vi "div3sum-tsk3.vi"() -> ()   [LabVIEW 2020]
panel:
  out "Numeric":dbl
  out "quotient":dbl
  out "remainder":dbl
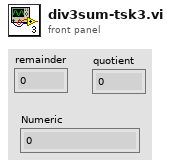
[diagram p1: front panel]
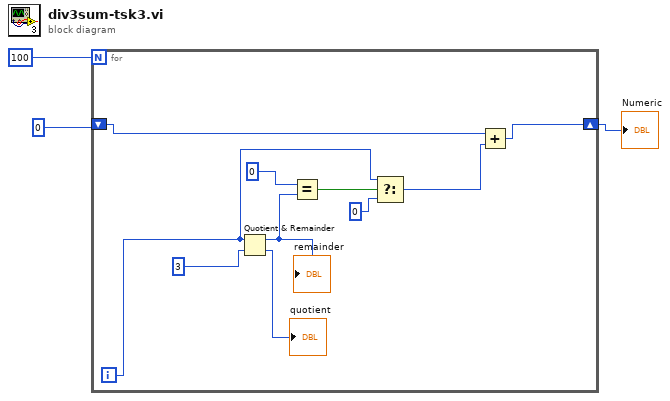
[diagram p0: block diagram]
diagram:
  n1 = for {
    N: 100 -> [_]
    shift-right: [w4] -> w1
    shift-left: 0 -> [w6]
    i -> [w7]
    n2 = Quotient & Remainder(x=w7, y=3) -> (x-y*floor(x/y)=w10:i32, floor(x/y)=→"quotient":i32)
    "remainder" <- w10
    n3 = Equal?(x=0, y=w10) -> (x = y?=w9:bool)
    n4 = Select(t=w7, s=w9, f=0) -> (s? t:f=w5:i32)
    n5 = Add(x=w6, y=w5) -> (x+y=w4:i32)
  }
  "Numeric" <- w1
